vi "svfa_Build Spectrum Info (NxM) (Dual).vi"(0 "stimulus signals X [EUx]":waveform(dbl)[](array[waveform]), 1 "processing control":T7(ring), 5 "response signals Y [EUy]":waveform(dbl)[](array[waveform]), 7 "window":T8=1 items=["None"=0, "Hanning"=1, "Hamming"=2, "Blackman-Harris"=3, "Exact Blackman"=4, "Blackman"=5, "Flat Top"=6, "4 Term B-Harris "=7, "7 Term B-Harris"=8, "Low Sidelobe"=9, "Force - Exponential"=10, "Blackman Nuttall"=11, "Triangle"=30, "Bartlett-Hanning"=31, "Bohman"=32, "Parzen"=33, "Welch"=34, "Kaiser"=60, "Dolph-Chebyshev"=61, "Gaussian"=62], 9 "window size":i32, 11 "error in (no error)":errorcluster, 12 "spectrum type":T3=enum."Frequency Response [Complex]", 13 "x-axis units":u16(ring)=1 items=["time"=0, "frequency"=1, "quefrency"=2, "revolutions"=3, "order"=4, "rpm"=11], 14 "spectra info in":T1[][](array[typedef]) {"x-axis units" items=["Time (s)"=0, "Frequency-CB (Hz)"=1, "Frequency-CPB (Hz)"=1248, "Frequency-Arbitrary (Hz)"=2357, "Quefrency (s)"=2, "Revolutions (rev)"=3, "Order"=4, "Speed (RPM)"=11, "Speed (rad/s)"=21, "Index"=65535]; "weighting filter" items=["Linear", "A-weighting", "B-weighting", "C-weighting", "ITU-R 468-4", "Dolby", "CCITT", "C-message", "Wb", "Wc", "Wd", "We", "Wf", "Wh", "Wj", "Wk", "Wm", "AES17 20 kHz lowpass", "AES17 40 kHz lowpass", "AES17 20 kHz highpass", "AES17 40 kHz highpass"]; "dB reference [EU]" format="%.2f"; "engineering units" items=["custom..."=0, "V"=1, "A"=21, "C"=30, "pC"=31, "s"=32, "-"=29, "Pa"=2, "N"=20, "g"=3, "m/s^2"=4, "m/s"=5, "m"=6, "mm/s"=12, "mm"=13, "micron/s"=14, "micron"=15, "in/s^2"=7, "in/s"=8, "in"=9, "mil/s"=10, "mil"=11, "rad/s^2"=16, "rad/s"=17, "rad"=18, "deg/s^2"=26, "deg/s"=27, "deg"=28, "RPM"=22, "cycle/s^2"=23, "Hz"=24, "cycle"=25, "strain"=19]; "spectral info"."window" items=["None "=0, "Hanning"=1, "Hamming"=2, "Blackman-Harris"=3, "Exact Blackman"=4, "Blackman"=5, "Flat Top"=6, "4 Term B-Harris "=7, "7 Term B-Harris"=8, "Low Sidelobe"=9, "Force - Exponential"=10, "Gaussian"=62]}) -> (3 "dup processing control":T7(ring), 4 "dup stimulus signals X [EUx]":waveform(dbl)[](array[waveform]), 6 "response signals Y [EUy]":waveform(dbl)[](array[waveform]), 10 "spectra info out":T1[][](array[typedef]) {"x-axis units" items=["Time (s)"=0, "Frequency-CB (Hz)"=1, "Frequency-CPB (Hz)"=1248, "Frequency-Arbitrary (Hz)"=2357, "Quefrency (s)"=2, "Revolutions (rev)"=3, "Order"=4, "Speed (RPM)"=11, "Speed (rad/s)"=21, "Index"=65535]; "weighting filter" items=["Linear", "A-weighting", "B-weighting", "C-weighting", "ITU-R 468-4", "Dolby", "CCITT", "C-message", "Wb", "Wc", "Wd", "We", "Wf", "Wh", "Wj", "Wk", "Wm", "AES17 20 kHz lowpass", "AES17 40 kHz lowpass", "AES17 20 kHz highpass", "AES17 40 kHz highpass"]; "dB reference [EU]" format="%.2f"; "engineering units" items=["custom..."=0, "V"=1, "A"=21, "C"=30, "pC"=31, "s"=32, "-"=29, "Pa"=2, "N"=20, "g"=3, "m/s^2"=4, "m/s"=5, "m"=6, "mm/s"=12, "mm"=13, "micron/s"=14, "micron"=15, "in/s^2"=7, "in/s"=8, "in"=9, "mil/s"=10, "mil"=11, "rad/s^2"=16, "rad/s"=17, "rad"=18, "deg/s^2"=26, "deg/s"=27, "deg"=28, "RPM"=22, "cycle/s^2"=23, "Hz"=24, "cycle"=25, "strain"=19]; "spectral info"."window" items=["None "=0, "Hanning"=1, "Hamming"=2, "Blackman-Harris"=3, "Exact Blackman"=4, "Blackman"=5, "Flat Top"=6, "4 Term B-Harris "=7, "7 Term B-Harris"=8, "Low Sidelobe"=9, "Force - Exponential"=10, "Gaussian"=62]}, 15 "error out":errorcluster)   [LabVIEW 2017]
uses:
  <vilib>/addons/_NISVFA/_Shared subVIs/Controls/svc_Spectrum Info.ctl
  <vilib>/addons/_NISVFA/_Shared subVIs/Controls/svc_X-Axis Units.ctl
  <vilib>/addons/_NISVFA/_Shared subVIs/Controls/svc_Spectrum Type.ctl
  <vilib>/addons/_NISVFA/_Shared subVIs/Controls/svc_Engineering Units Text Ring.ctl
  <vilib>/addons/_NISVFA/_Shared subVIs/Controls/svc_Weighting Filter Text Ring.ctl
  <vilib>/addons/_NISVFA/_Shared subVIs/Controls/svc_Complimentary Spectrum Units.ctl
  <vilib>/addons/_NISVFA/_Shared subVIs/Controls/svc_Window [Dual FFT].ctl
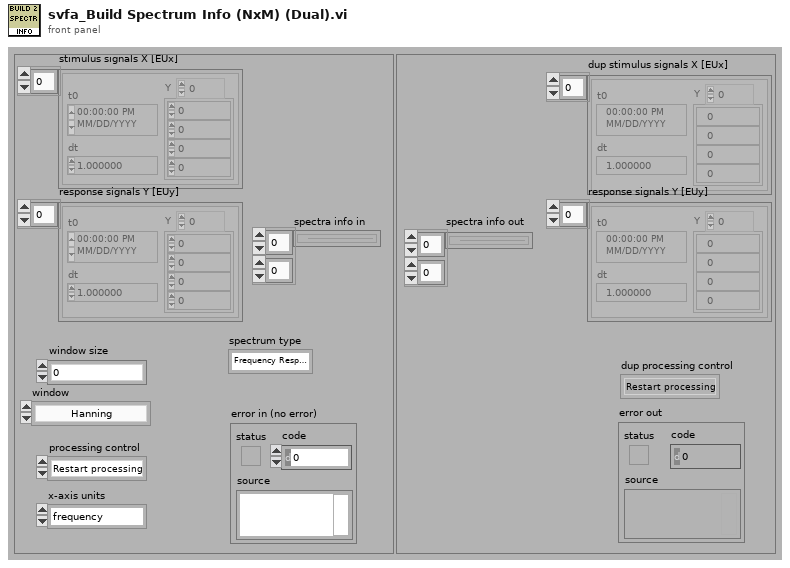
[diagram p1: front panel]
types:
  T1 = typedef "svc_Spectrum Info.ctl" = cluster{"channel name":string, "description":string, "x-axis units":T2, "spectral info":cluster{"spectrum type":T3, "linear/dB":enum16{"linear", "dB"}, "window":u16, "window size":i32, "FFT size":i32}, "engineering units":T4, "custom label":string, "dB reference [EU]":dbl, "peak units":enum16{"rms", "peak", "peak-peak"}, "weighting filter":T5, "spectral density?":bool, "unit label":string, "spectrum skewed?":bool, "complimentary spectrum units":T6}
  T2 = typedef "svc_X-Axis Units.ctl" = u16
  T3 = typedef "svc_Spectrum Type.ctl" = enum16{"FFT Spectrum [complex]", "Amplitude [Magnitude]", "Power [Magnitude^2]", "Cross Spectrum [complex]", "Frequency Response [Complex]"}
  T4 = typedef "svc_Engineering Units Text Ring.ctl" = u16
  T5 = typedef "svc_Weighting Filter Text Ring.ctl" = u16
  T6 = typedef "svc_Complimentary Spectrum Units.ctl" = enum16{"none", "radians", "degrees", "cycles", "imaginary"}
  T7 = enum16{"Restart processing", "Continue processing", "Skip processing"}
  T8 = typedef "svc_Window [Dual FFT].ctl" = u32
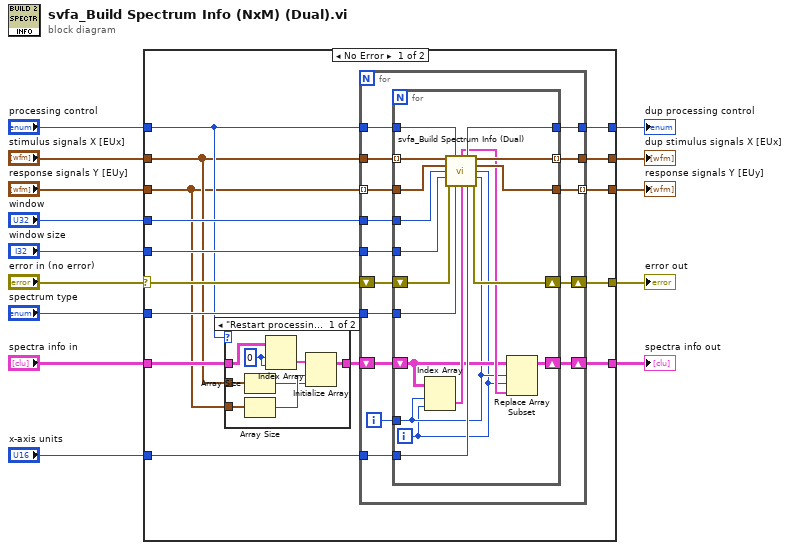
[diagram p0: block diagram]
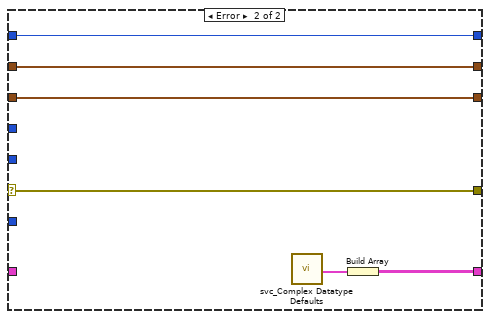
[diagram p3: hidden frame]
diagram:
  n1 = case shown="No Error" "error in (no error)" {
    selector: "error in (no error)" -> [w26 w77]
    tunnel: [w21 w72] -> w3
    tunnel: "stimulus signals X [EUx]" -> [w16 w76]
    tunnel: [w29 w76] -> w7
    tunnel: [w25 w77] -> w13
    tunnel: "response signals Y [EUy]" -> [w15 w75]
    tunnel: [w28 w75] -> w6
    tunnel: "spectrum type" -> [w27 _]
    tunnel: "window" -> [w24 _]
    tunnel: "window size" -> [w23 _]
    tunnel: "processing control" -> [w19 w74]
    tunnel: [w22 w74] -> w5
    tunnel: "spectra info in" -> [w18 _]
    tunnel: "x-axis units" -> [w20 _]
    frame No Error {
      n2 = case shown="\"Restart processing\"" w19 {
        tunnel: [w36 w38] -> w17
        tunnel: w18 -> [w37 w38]
        tunnel: w16 -> [w33 _]
        tunnel: w15 -> [w32 _]
        frame "Restart processing" {
          w34 = 0 ("index (row)")
          n3 = Array Size(array=w33) -> (size(s)=w30:i32)
          n4 = Array Size(array=w32) -> (size(s)=w31:i32)
          n5 = Index Array(array=w37, index (row)=w34, index (col)=w34) -> (element=w35:T1)
          n6 = Initialize Array(w35, w31, w30) -> (w36:T1[][])
        }
        frame "Continue processing", Default {
        }
      }
      n7 = for {
        tunnel: w16 -> [w53]
        tunnel: [w52] -> w29
        tunnel: w15 -> [w51] mode=indexing
        tunnel: [w50] -> w28 mode=indexing
        tunnel: w27 -> [w49]
        tunnel: w24 -> [w46]
        tunnel: w23 -> [w45]
        tunnel: w19 -> [w44]
        tunnel: [w43] -> w22
        shift-right: [w47] -> w25
        shift-left: w26 -> [w48]
        tunnel: w20 -> [w40]
        shift-right: [w41] -> w21
        shift-left: w17 -> [w42]
        i -> [w39]
        n8 = for {
          tunnel: w53 -> [w68] mode=indexing
          tunnel: [w66] -> w52 mode=indexing
          tunnel: w51 -> [w69]
          tunnel: [w65] -> w50
          tunnel: w49 -> [w67]
          tunnel: w46 -> [w71]
          tunnel: w45 -> [w70]
          tunnel: w44 -> [w64]
          tunnel: [w63] -> w43
          shift-right: [w61] -> w47
          shift-left: w48 -> [w62]
          tunnel: w40 -> [w60]
          shift-right: [w56] -> w41
          shift-left: w42 -> [w57]
          tunnel: w39 -> [w55]
          i -> [w54]
          n9 = Index Array(array=w57, index (row)=w55, index (col)=w54) -> (element=w59:T1)
          n10 = call <vilib>:"svfa_Build Spectrum Info (Dual).vi"("scaled signal  X [EU]"=w68, "processing control"=w64, "scaled signal  Y [EU]"=w69, "window"=w71, "x-channel index"=w54, "window size"=w70, "y-channel index"=w55, "error in (no error)"=w62, "spectrum type"=w67, "spectrum info in"=w59, "x-axis units"=w60) -> ("spectrum info out"=w58:T1, "dup processing control"=w63:T7, "dup scaled signal  X [EU]"=w66:waveform(dbl), "dup scaled signal  Y [EU]"=w65:waveform(dbl), "error out"=w61:errorcluster)
          n11 = Replace Array Subset(array=w57, new element=w58, index (row)=w55, index (col)=w54) -> (w56:T1[][])
        }
      }
    }
    frame Error {
      n12 = call <vilib>:"svc_Complex Datatype Defaults.vi"() -> ("empty array of spectrum info"=w73:T1[])  [unwired: 11 in, 8 out]
      n13 = Build Array(w73) -> (w72:T1[][])
    }
  }
  "spectra info out" <- w3
  "error out" <- w13
  "dup processing control" <- w5
  "dup stimulus signals X [EUx]" <- w7
  "response signals Y [EUy]" <- w6
